vi "Update Main GUI - Tabs.vi"(8 "error in":errorcluster, 10 "GUI Command":T1=enum."Initialise", 11 "Main GUI Refnum":refnum<vi>) -> (0 "error out":errorcluster)   [LabVIEW 2017, in "DTacq Plot Display Library.lvlib"]
uses:
  DTacq Plot Display Library.lvlib
  Typedefs/Graphical Interface Commands - Tabs--Enum.ctl
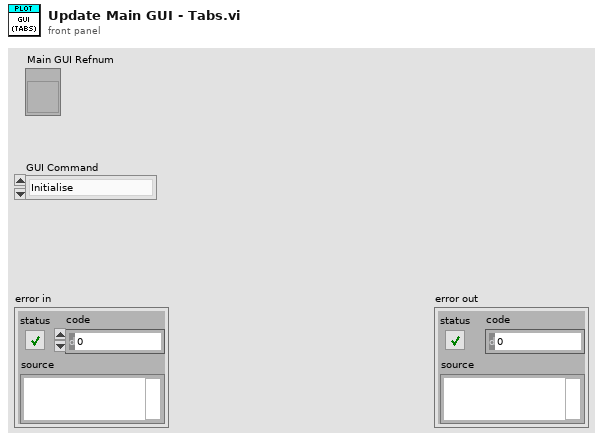
[diagram p1: front panel]
types:
  T1 = typedef "DTacq Plot Display Library.lvlib/Graphical Interface Commands - Tabs--Enum.ctl" = enum16{"Close GUI", "Initialise", "Add Tab", "Close Tab", "Update Buttons"}
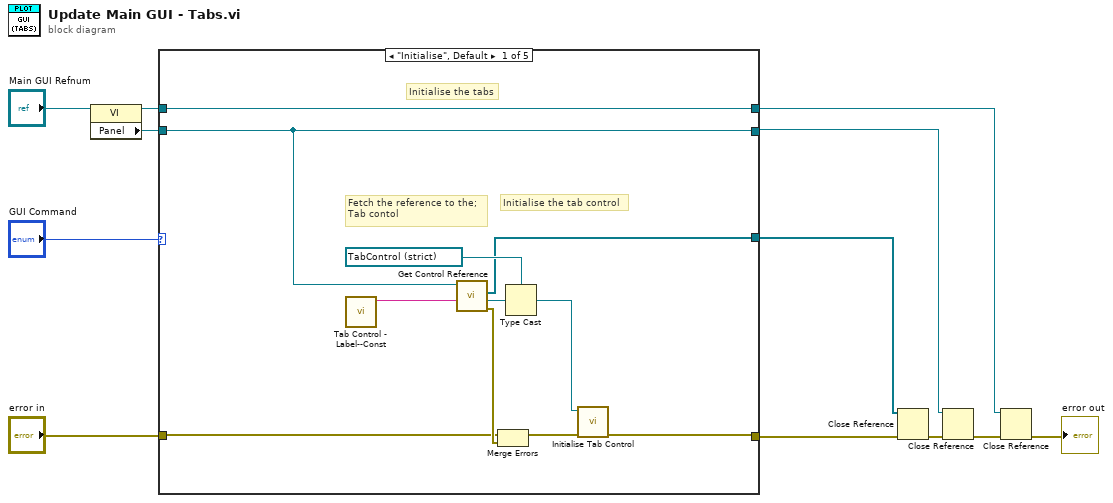
[diagram p0: block diagram]
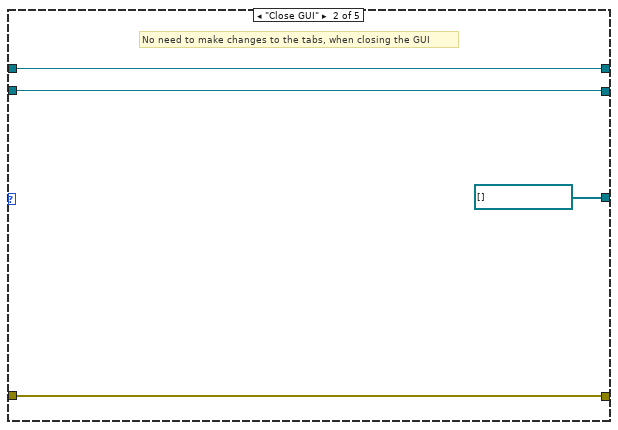
[diagram p2: hidden frame]
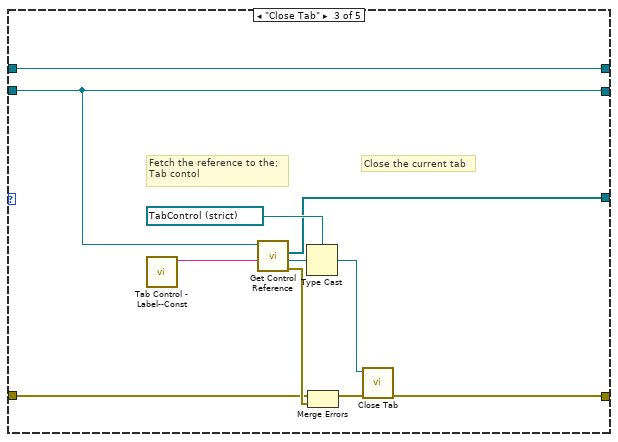
[diagram p3: hidden frame]
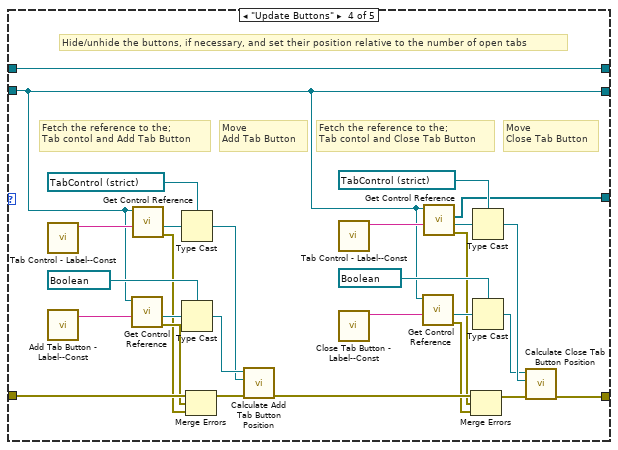
[diagram p4: hidden frame]
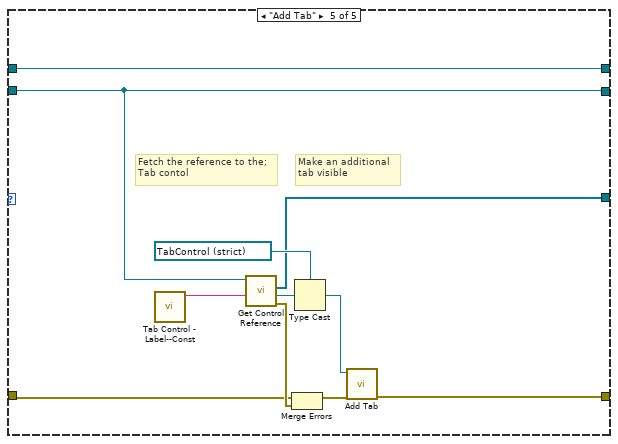
[diagram p5: hidden frame]
diagram:
  n1 = property class="VI"(reference="Main GUI Refnum") -> (reference out=w7:refnum<vi>, "Panel"=w8:refnum<vi>)  [unwired: 1 in, 1 out]
  n2 = case shown="\"Initialise\", Default" "GUI Command" {
    tunnel: "error in" -> [w14 w26 w29 w46 w67]
    tunnel: [w17 w25 w32 w48 w71] -> w10
    tunnel: [w19 w26 w38 w66 w77] -> w5
    tunnel: w8 -> [w17 w25 w32 w48 w71]
    tunnel: w7 -> [w16 w24 w31 w47 w70]
    tunnel: [w18 refnum<vi>[] [] ("Control References Array") w33 w49 w72] -> w6
    tunnel: [w16 w24 w31 w47 w70] -> w1
    frame "Initialise", Default {
      # "Initialise the tab control"
      # "Initialise the tabs"
      # "Fetch the reference to the;\nTab contol"
      n3 = call "Tab Control - Label--Const.vi"() -> ("Tab Control Label"=w23:string)  [unwired: 11 in]
      n4 = call "Get Control Reference.vi"("Control Label"=w23, "Front Panel Reference In"=w17) -> ("error out"=w15:errorcluster, "Selected Control Reference"=w21:refnum<vi>, "Control References Array"=w18:refnum<vi>[])  [unwired: 6 in, 1 out]
      n5 = Merge Errors(w14, w15) -> (w13:errorcluster)
      n6 = Type Cast(type=refnum<vi> refnum ("Tab Control Reference"), x=w21) -> (*(type *) &x=w20:refnum<vi>)
      n7 = call "Initialise Tab Control.vi"("error in"=w13, "Tab Control Reference In"=w20) -> ("error out"=w19:errorcluster)  [unwired: 9 in]
    }
    frame "Close GUI" {
      # "No need to make changes to the tabs, when closing the GUI"
    }
    frame "Close Tab" {
      # "Close the current tab"
      # "Fetch the reference to the;\nTab contol"
      n8 = call "Tab Control - Label--Const.vi"() -> ("Tab Control Label"=w37:string)  [unwired: 11 in]
      n9 = call "Get Control Reference.vi"("Control Label"=w37, "Front Panel Reference In"=w32) -> ("error out"=w30:errorcluster, "Selected Control Reference"=w35:refnum<vi>, "Control References Array"=w33:refnum<vi>[])  [unwired: 6 in, 1 out]
      n10 = Type Cast(type=refnum<vi> refnum ("Tab Control Reference"), x=w35) -> (*(type *) &x=w34:refnum<vi>)
      n11 = Merge Errors(w29, w30) -> (w28:errorcluster)
      n12 = call "Close Tab.vi"("error in"=w28, "Tab Control Reference In"=w34) -> ("error out"=w38:errorcluster)  [unwired: 8 in, 1 out]
    }
    frame "Update Buttons" {
      # "Hide/unhide the buttons, if necessary, and set their position relative to the number of open tabs"
      # "Move\nClose Tab Button"
      # "Move\nAdd Tab Button"
      # "Fetch the reference to the;\nTab contol and Add Tab Button"
      # "Fetch the reference to the;\nTab contol and Close Tab Button"
      n13 = call "Tab Control - Label--Const.vi"() -> ("Tab Control Label"=w57:string)  [unwired: 11 in]
      n14 = call "Add Tab Button - Label--Const.vi"() -> ("Add Tab Control Label"=w50:string)  [unwired: 11 in]
      n15 = call "Get Control Reference.vi"("Control Label"=w50, "Front Panel Reference In"=w48) -> ("error out"=w45:errorcluster, "Selected Control Reference"=w54:refnum<vi>)  [unwired: 6 in, 2 out]
      n16 = call "Get Control Reference.vi"("Control Label"=w57, "Front Panel Reference In"=w48) -> ("error out"=w43:errorcluster, "Selected Control Reference"=w55:refnum<vi>)  [unwired: 6 in, 2 out]
      n17 = Type Cast(type=refnum<vi> refnum ("Tab Control Reference"), x=w55) -> (*(type *) &x=w51:refnum<vi>)
      n18 = Type Cast(type=refnum<vi> refnum ("Close Tab Button Reference"), x=w54) -> (*(type *) &x=w52:refnum<vi>)
      n19 = Merge Errors(w46, w45, w43) -> (w44:errorcluster)
      n20 = call "Calculate Add Tab Button Position.vi"("error in"=w44, "Tab Control Reference In"=w51, "Add Tab Button Reference In"=w52) -> ("error out"=w42:errorcluster)  [unwired: 5 in, 3 out]
      n21 = call "Tab Control - Label--Const.vi"() -> ("Tab Control Label"=w65:string)  [unwired: 11 in]
      n22 = call "Close Tab Button - Label--Const.vi"() -> ("Close Tab Control Label"=w61:string)  [unwired: 11 in]
      n23 = call "Get Control Reference.vi"("Control Label"=w61, "Front Panel Reference In"=w48) -> ("error out"=w40:errorcluster, "Selected Control Reference"=w60:refnum<vi>)  [unwired: 6 in, 2 out]
      n24 = call "Get Control Reference.vi"("Control Label"=w65, "Front Panel Reference In"=w48) -> ("error out"=w41:errorcluster, "Selected Control Reference"=w63:refnum<vi>, "Control References Array"=w49:refnum<vi>[])  [unwired: 6 in, 1 out]
      n25 = Merge Errors(w42, w41, w40) -> (w39:errorcluster)
      n26 = Type Cast(type=refnum<vi> refnum ("Tab Control Reference"), x=w63) -> (*(type *) &x=w62:refnum<vi>)
      n27 = Type Cast(type=refnum<vi> refnum ("Close Tab Button Reference"), x=w60) -> (*(type *) &x=w58:refnum<vi>)
      n28 = call "Calculate Close Tab Button Position.vi"("error in"=w39, "Tab Control Reference In"=w62, "Close Tab Button Reference In"=w58) -> ("error out"=w66:errorcluster)  [unwired: 5 in, 3 out]
    }
    frame "Add Tab" {
      # "Make an additional\ntab visible"
      # "Fetch the reference to the;\nTab contol"
      n29 = call "Tab Control - Label--Const.vi"() -> ("Tab Control Label"=w76:string)  [unwired: 11 in]
      n30 = call "Get Control Reference.vi"("Control Label"=w76, "Front Panel Reference In"=w71) -> ("error out"=w68:errorcluster, "Selected Control Reference"=w74:refnum<vi>, "Control References Array"=w72:refnum<vi>[])  [unwired: 6 in, 1 out]
      n31 = Merge Errors(w67, w68) -> (w69:errorcluster)
      n32 = Type Cast(type=refnum<vi> refnum ("Tab Control Reference"), x=w74) -> (*(type *) &x=w73:refnum<vi>)
      n33 = call "Add Tab.vi"("error in"=w69, "Tab Control Reference In"=w73) -> ("error out"=w77:errorcluster)  [unwired: 8 in, 1 out]
    }
  }
  n34 = Close Reference(reference=w6, error in (no error)=w5) -> (error out=w4:errorcluster)
  n35 = Close Reference(reference=w10, error in (no error)=w4) -> (error out=w3:errorcluster)
  n36 = Close Reference(reference=w1, error in (no error)=w3) -> (error out=→"error out":errorcluster)
